vi "Signalverlaeufe in Graphen Umladen.vi"(4 "Deviation":sgl[](array[numeric]), 6 "Mittelwertdaten":sgl[][](array[numeric]), 8 "Gas-Auswahl":T1, 9 "t0":timestamp, 11 "Werte":sgl[][](array[numeric])) -> (0 "Konzentration":sgl, 2 "Mittelwert":waveform(dbl), 3 "Waveform":waveform(dbl), 5 "aktuelle Mittelwert":sgl, 7 "Deviation":sgl)   [LabVIEW 2020, in "Grafik.lvlib"]
uses:
  Grafik.lvlib
  Visualisierungs Elemente/Auswahlfeld.ctl
  FT-IR/FGV FT-IR Aktionen.ctl
  FT-IR/FT-IR.lvlib
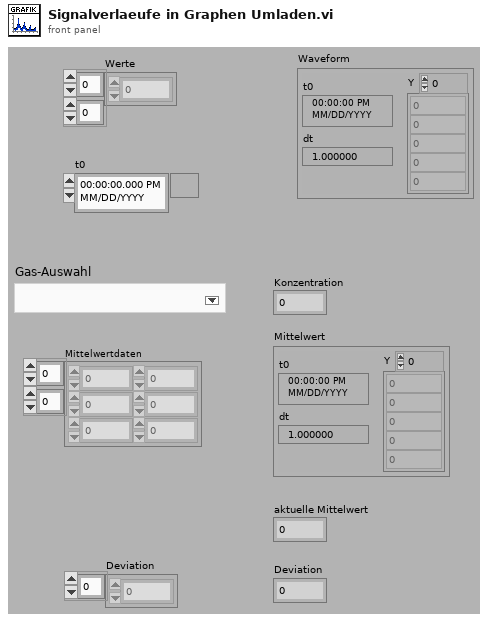
[diagram p1: front panel]
types:
  T1 = typedef "Auswahlfeld.ctl" = u16
  T2 = typedef "FT-IR.lvlib/FGV FT-IR Aktionen.ctl" = enum16{"lesen", "NOG setzen", "NOS setzen", "Initialisieren", "speichern", "ALLES setzen", "FT-IR Spektrum loggen", "Komm Stoppen", "Spektrum LogKonfig"}
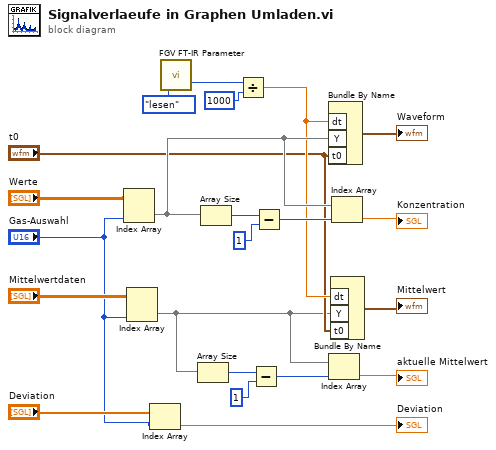
[diagram p0: block diagram]
diagram:
  n1 = Index Array(array="Werte", index (col)="Gas-Auswahl") -> (element=w16:sgl[])  [unwired: 1 in]
  n2 = Index Array(array="Mittelwertdaten", index (col)="Gas-Auswahl") -> (element=w7:sgl[])  [unwired: 1 in]
  n3 = Index Array(array="Deviation", index="Gas-Auswahl") -> (element=→"Deviation":sgl)
  n4 = call "FGV FT-IR Parameter.vi"("Aktion"=FGV_FT-IR_Aktionen."lesen") -> ("Zykluszeit Messdatenverteiler"=w3:u32)  [unwired: 11 in, 7 out]
  n5 = Array Size(array=w7) -> (size(s)=w9:i32)
  n6 = Array Size(array=w16) -> (size(s)=w21:i32)
  n7 = Divide(x=w3, y=u32 1000) -> (x/y=w14:dbl)
  n8 = Subtract(x=w9, y=1) -> (x-y=w11:i32)
  n9 = Subtract(x=w21, y=1) -> (x-y=w19:i32)
  n10 = Bundle By Name("dt"=w14, "Y"=w16, "t0"="t0") -> (→"Waveform":waveform(sgl))  [unwired: 1 out]
  n11 = Index Array(array=w7, index=w11) -> (element=→"aktuelle Mittelwert":sgl)
  n12 = Bundle By Name("dt"=w14, "Y"=w7, "t0"="t0") -> (→"Mittelwert":waveform(sgl))  [unwired: 1 out]
  n13 = Index Array(array=w16, index=w19) -> (element=→"Konzentration":sgl)
